vi "Mark Module Used.vi"(8 "error in":errorcluster, 10 "validation information in":T1, 11 "module path":string) -> (0 "error out":errorcluster, 2 "validation information out":T1)   [LabVIEW 2020, in "Routing and Faulting Scripting.lvlib"]
uses:
  Routing and Faulting Scripting.lvlib
  Validation Information.ctl
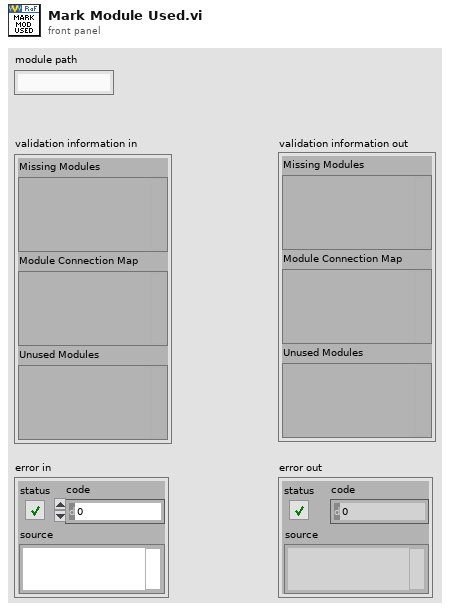
[diagram p1: front panel]
types:
  T1 = typedef "Routing and Faulting Scripting.lvlib/Validation Information.ctl" = cluster{"Missing Modules":variant, "Module Connection Map":variant, "Unused Modules":variant}
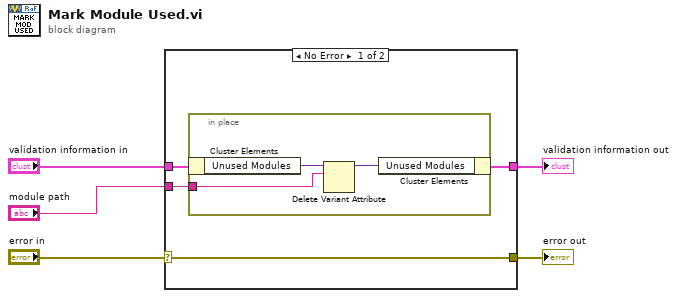
[diagram p0: block diagram]
diagram:
  n1 = case shown="No Error" "error in" {
    selector: "error in" -> [w6 w13]
    tunnel: "validation information in" -> [w9 w14]
    tunnel: "module path" -> [w8 _]
    tunnel: [w7 w14] -> w3
    tunnel: [w6 w13] -> w1
    frame No Error {
      n2 = in-place {
        in-place-border: w8 -> [w10]
        n3 = in-place-cluster #1(w9) -> ("Unused Modules"=w12:variant)
        n4 = Delete Variant Attribute(6:w10, 7:w12) -> (3:w11:variant)  [unwired: 1 in, 2 out]
        n5 = in-place-cluster #1("Unused Modules"=w11) -> (w7:T1)
      }
    }
    frame Error {
    }
  }
  "error out" <- w1
  "validation information out" <- w3
